vi "Create Pattern Script(one timeset).vi"(7 "Notes":string, 9 "Pin States":T1[](array[typedef]), 10 "timeset name":string="-", 11 "opcode":string) -> (3 "string out":string)   [LabVIEW 2018, in "Protocol Interface.lvlib" / "Protocol Interface.lvclass"]
uses:
  Protocol Interface.lvclass
  Pin State.ctl
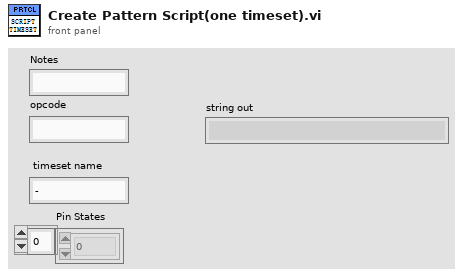
[diagram p1: front panel]
types:
  T1 = typedef "Protocol Interface.lvlib/Protocol Interface.lvclass/Pin State.ctl" = enum16{"0", "1", "L", "H", "X", "V", "D", "M"}
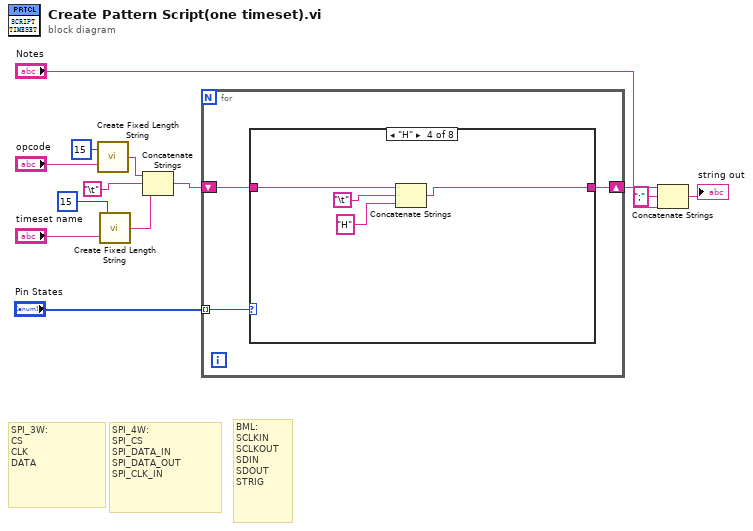
[diagram p0: block diagram]
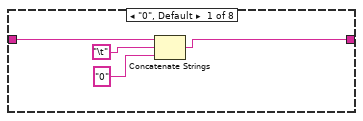
[diagram p2: hidden frame]
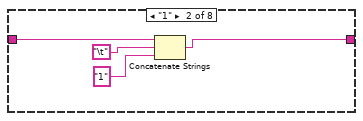
[diagram p3: hidden frame]
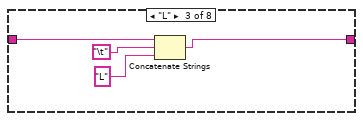
[diagram p4: hidden frame]
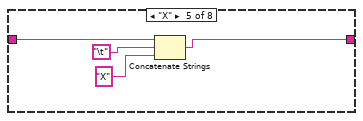
[diagram p5: hidden frame]
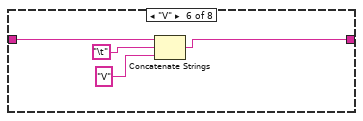
[diagram p6: hidden frame]
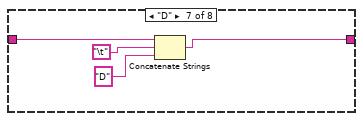
[diagram p7: hidden frame]
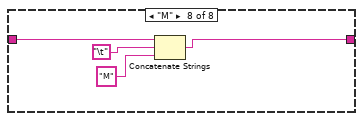
[diagram p8: hidden frame]
diagram:
  # "SPI_3W:\nCS\nCLK\nDATA"
  # "SPI_4W:\nSPI_CS\nSPI_DATA_IN\nSPI_DATA_OUT\nSPI_CLK_IN"
  # "BML:\nSCLKIN\nSCLKOUT\nSDIN\nSDOUT\nSTRIG"
  n1 = call "Create Fixed Length String.vi"("String"="opcode", "Length"=u32 15) -> ("String out"=w4:string)
  n2 = call "Create Fixed Length String.vi"("String"="timeset name", "Length"=u32 15) -> ("String out"=w1:string)
  n3 = Concatenate Strings(w4, "\t", w1) -> (w12:string)
  n4 = for {
    tunnel: "Pin States" -> [w16] mode=indexing
    shift-right: [w14] -> w11
    shift-left: w12 -> [w15]
    n5 = case shown="\"H\"" w16 {
      tunnel: w15 -> [w20 w24 w28 w32 w36 w40 w44 w48]
      tunnel: [w17 w21 w25 w29 w33 w37 w41 w45] -> w14
      frame "0", Default {
        n6 = Concatenate Strings(w20, "\t", "0") -> (w17:string)
      }
      frame "1" {
        n7 = Concatenate Strings(w24, "\t", "1") -> (w21:string)
      }
      frame "L" {
        n8 = Concatenate Strings(w28, "\t", "L") -> (w25:string)
      }
      frame "H" {
        n9 = Concatenate Strings(w32, "\t", "H") -> (w29:string)
      }
      frame "X" {
        n10 = Concatenate Strings(w36, "\t", "X") -> (w33:string)
      }
      frame "V" {
        n11 = Concatenate Strings(w40, "\t", "V") -> (w37:string)
      }
      frame "D" {
        n12 = Concatenate Strings(w44, "\t", "D") -> (w41:string)
      }
      frame "M" {
        n13 = Concatenate Strings(w48, "\t", "M") -> (w45:string)
      }
    }
  }
  n14 = Concatenate Strings(w11, ";" ("string"), "Notes") -> (→"string out":string)
